vi "1.4.vi"() -> ()   [LabVIEW 2017]
panel:
  out "sin":dbl
  in  "graden":dbl
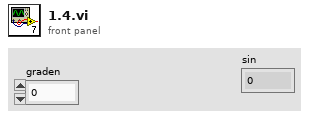
[diagram p1: front panel]
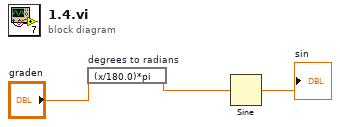
[diagram p0: block diagram]
diagram:
  n1 = expression code="(x/180.0)*pi" "degrees to radians"("graden") -> (w2:dbl)
  n2 = Sine(x=w2) -> (sin(x)=→"sin":dbl)
